vi "LIDAR V6 FPGA Main.vi"() -> ()   [LabVIEW 2013]
uses:
  Controls/FPGA Nain State.ctl
  Controls/Scan Format Typedaf.ctl
  <vilib>/Platform/TimedLoop/XDataNode/timing_clust.ctl
  <vilib>/Platform/TimedLoop/XDataNode/nitl_modes.ctl
  <vilib>/Platform/TimedLoop/XDataNode/wakeup.ctl
  Controls/Algorithm State.ctl
  <instrlib>/_niInstr/DSP/v1/Shared/Public/IQ Data.ctl
  <vilib>/rvi/Emulation/niFpgaSctlEmulationGetInTimedLoop.vi
  <vilib>/rvi/Emulation/niFpgaEmulationReportErrorSimple.vi
  <vilib>/rvi/Emulation/niFpgaGetClockAttributes.vi
  <vilib>/rvi/FIFO/Fifo_Resource/nirvififoEmulationReadFpgaImpl.vi
  <vilib>/rvi/DataTransferAndStorage/Container/Common/niFpgaContainerGetUniqueNameForEmu.vi
  <vilib>/rvi/eio/common/nirviEmuTemplateMethod_errors.vi
  <vilib>/rvi/Emulation/niFpgaCriticalErrorInLSC.vi
  <vilib>/rvi/Emulation/niFpgaProcessEmulError.vi
  LIDAR V2 Globals.vi
  <vilib>/rvi/FIFO/Fifo_Resource/nirvififoEmulationWriteFpgaImpl.vi
  <instrlib>/_niInstr/DSP/v1/FPGA/Private/Fractional Decimator/Fractional Decimator - 1 spc - 2x oc.vi
  <vilib>/rvi/interface/RandomDataEmulation/nirviRandomDataFPGAFIFO.vi
  <vilib>/rvi/interface/RandomDataEmulation/niFpgaRandomDataHandleErrors.vi
  <vilib>/Platform/TimedLoop/XDataNode/XDataNode.xnode
  <vilib>/rvi/DataTransferAndStorage/Container/XNode/niFpgaContainer.xnode
  <vilib>/rvi/FIFO/Fifo_Resource/nirvififoEmulationRead.vi
  <vilib>/eio/EIONode/EIONode.xnode
  <vilib>/rvi/FIFO/Fifo_Resource/nirvififoEmulationWrite.vi
  <vilib>/rvi/FXPMathLib/FxpInterpret/XNode/nifxpmath_Interpret.xnode
  <vilib>/rvi/interface/RandomDataEmulation/nirviRandomDataFpgaReadWriteTemplate.vi
  <vilib>/Platform/TimedLoop/XDataNode/XDNodeRunTimeDep.lvlib
  <instrlib>/_niInstr/DSP/v1/FPGA/niInstr DSP v1 FPGA.lvlib
  <instrlib>/_niInstr/DSP/v1/Shared/niInstr DSP v1 Shared.lvlib
panel:
  out "AI 0":i16
  in  "delay":fxp<+/-,16,0>
  in  "output sample rate":fxp<+,48,1>=0.799994660000003 format="%#.10g"
  in  "MaxStartSample":u8
  in  "LedScanDebEn":bool
  in  "ActiveLedIndexDeb":u16
  in  "10thIndexDeb":u8
  in  "PulseUpClck":u16=3
  in  "PulseWaitClck":u16=40
  in  "AO Trig":bool
  in  "Devider":u8=3
  in  "PFI3":bool
  in  "PFI2":bool
  in  "User Command Commit":bool
  in  "User Command":u8
  out "User Command Idle":bool
  out "User Command Status":u8
  in  "User Data 0":u8
  in  "User Data 1":u8
  out "User Error":bool
  out "Configured?":bool
  in  "MemDebStart":u32
  in  "MemDebEnd":u32
  in  "ReadMemSel":bool
  in  "ReadMem":bool
  in  "NextLedEn":bool
  out "SimCoarsMaxIndex":u16
  out "SimFineMaxIndex":u16
  out "SimOut":i16
  out "SPI Idle":bool
  out "PLL Locked":bool
  in  "Clock":u8=1
  out "PLL Counter":i32
  in  "IO Module\\Apply Settings":bool
  out "LedAddress":u16
  in  "SingleCycle":bool
  in  "PulsePerLed":i16=199
  in  "ScanFormat":T1=enum."FullScanPerLed"
  in  "SamplingEnable":bool
  out "MainState":T2
  out "10thIndex":u8
  out "PulseIndex":i16
  in  "MemSel":bool
  in  "ActiveLedIndex":u16
  out "InitMem":bool
  out "PulseEnd":bool
  in  "SampPerPulse":u16=99
  out "IterReset":u16 format="%.0b"
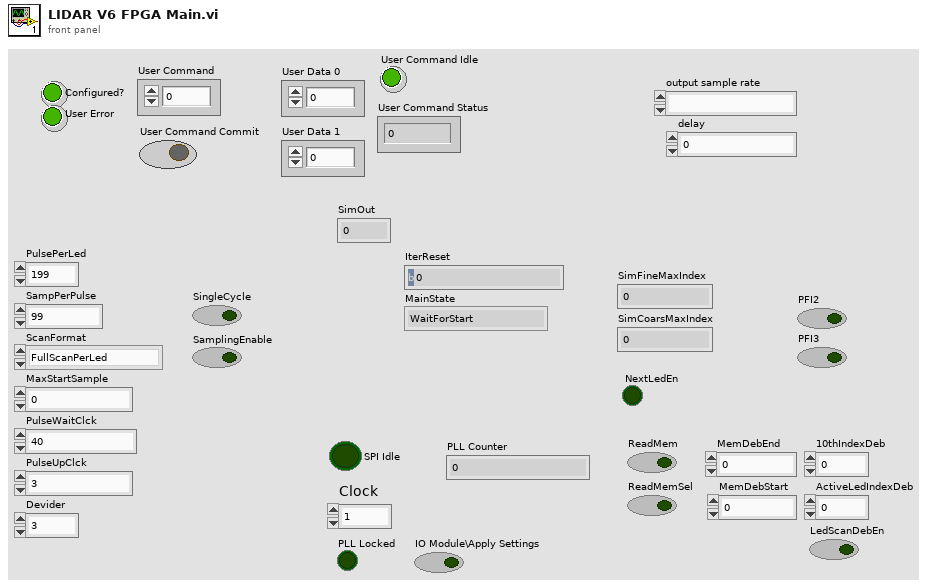
[diagram p1: front panel]
types:
  T1 = typedef "Scan Format Typedaf.ctl" = enum16{"1PulsePerLed", "FullScanPerLed"}
  T2 = typedef "FPGA Nain State.ctl" = enum16{"WaitForStart", "SetProcParams", "SelectActiveLed", "ActivatePulse", "WaitForPulseEnd", "WaitForAlgoStart", "SingleCycleEnd"}
  T3 = typedef "XDNodeRunTimeDep.lvlib/timing_clust.ctl" = cluster{"Expected End [f-1]":u64, "Actual End [f-1]":u64, "Finished Late? [f-1]":bool, "Expected End [i-1]":u64, "Actual End [i-1]":u64, "Finished Late? [i-1]":bool, "Expected Start [i]":u64, "Actual Start [i]":u64, "Expected Start [f]":u64, "Actual Start [f]":u64, "Source Name":string, "Structure Name":string, "Period":i64, "Deadline":i64, "Offset":i64, "Start":i64, "Priority":i32, "Timeout":i32, "Mode":T4, "Wakeup Reason":T5, "Error":errorcluster, "Source Type":string, "Secondary Source Type":string, "Global End Time":u64, "Global Start Time":u64, "Frame Duration":u64, "Iteration Duration":u64, "Assigned CPU":i32, "I/O Scan Engine Mode":u32}
  T4 = typedef "XDNodeRunTimeDep.lvlib/nitl_modes.ctl" = enum32{"No Change", "Process missed periods, maintain original phase", "Discard missed periods, maintain original phase", "Process missed periods, ignore original phase", "Discard missed periods, ignore original phase"}
  T5 = typedef "XDNodeRunTimeDep.lvlib/wakeup.ctl" = enum32{"Normal", "Aborted", "Asynchronous wakeup", "Timing source error", "Timed loop error", "Timeout"}
  T6 = typedef "niInstr DSP v1 Shared.lvlib/IQ Data.ctl" = cluster{"I":fxp<+/-,18,1>, "Q":fxp<+/-,18,1>, "overflow":bool}
  T7 = typedef "Algorithm State.ctl" = enum16{"WaitForStart", "GetNextSignalElement", "WaitForNextSignalElem", "MultWithSinc", "CalcMax"}
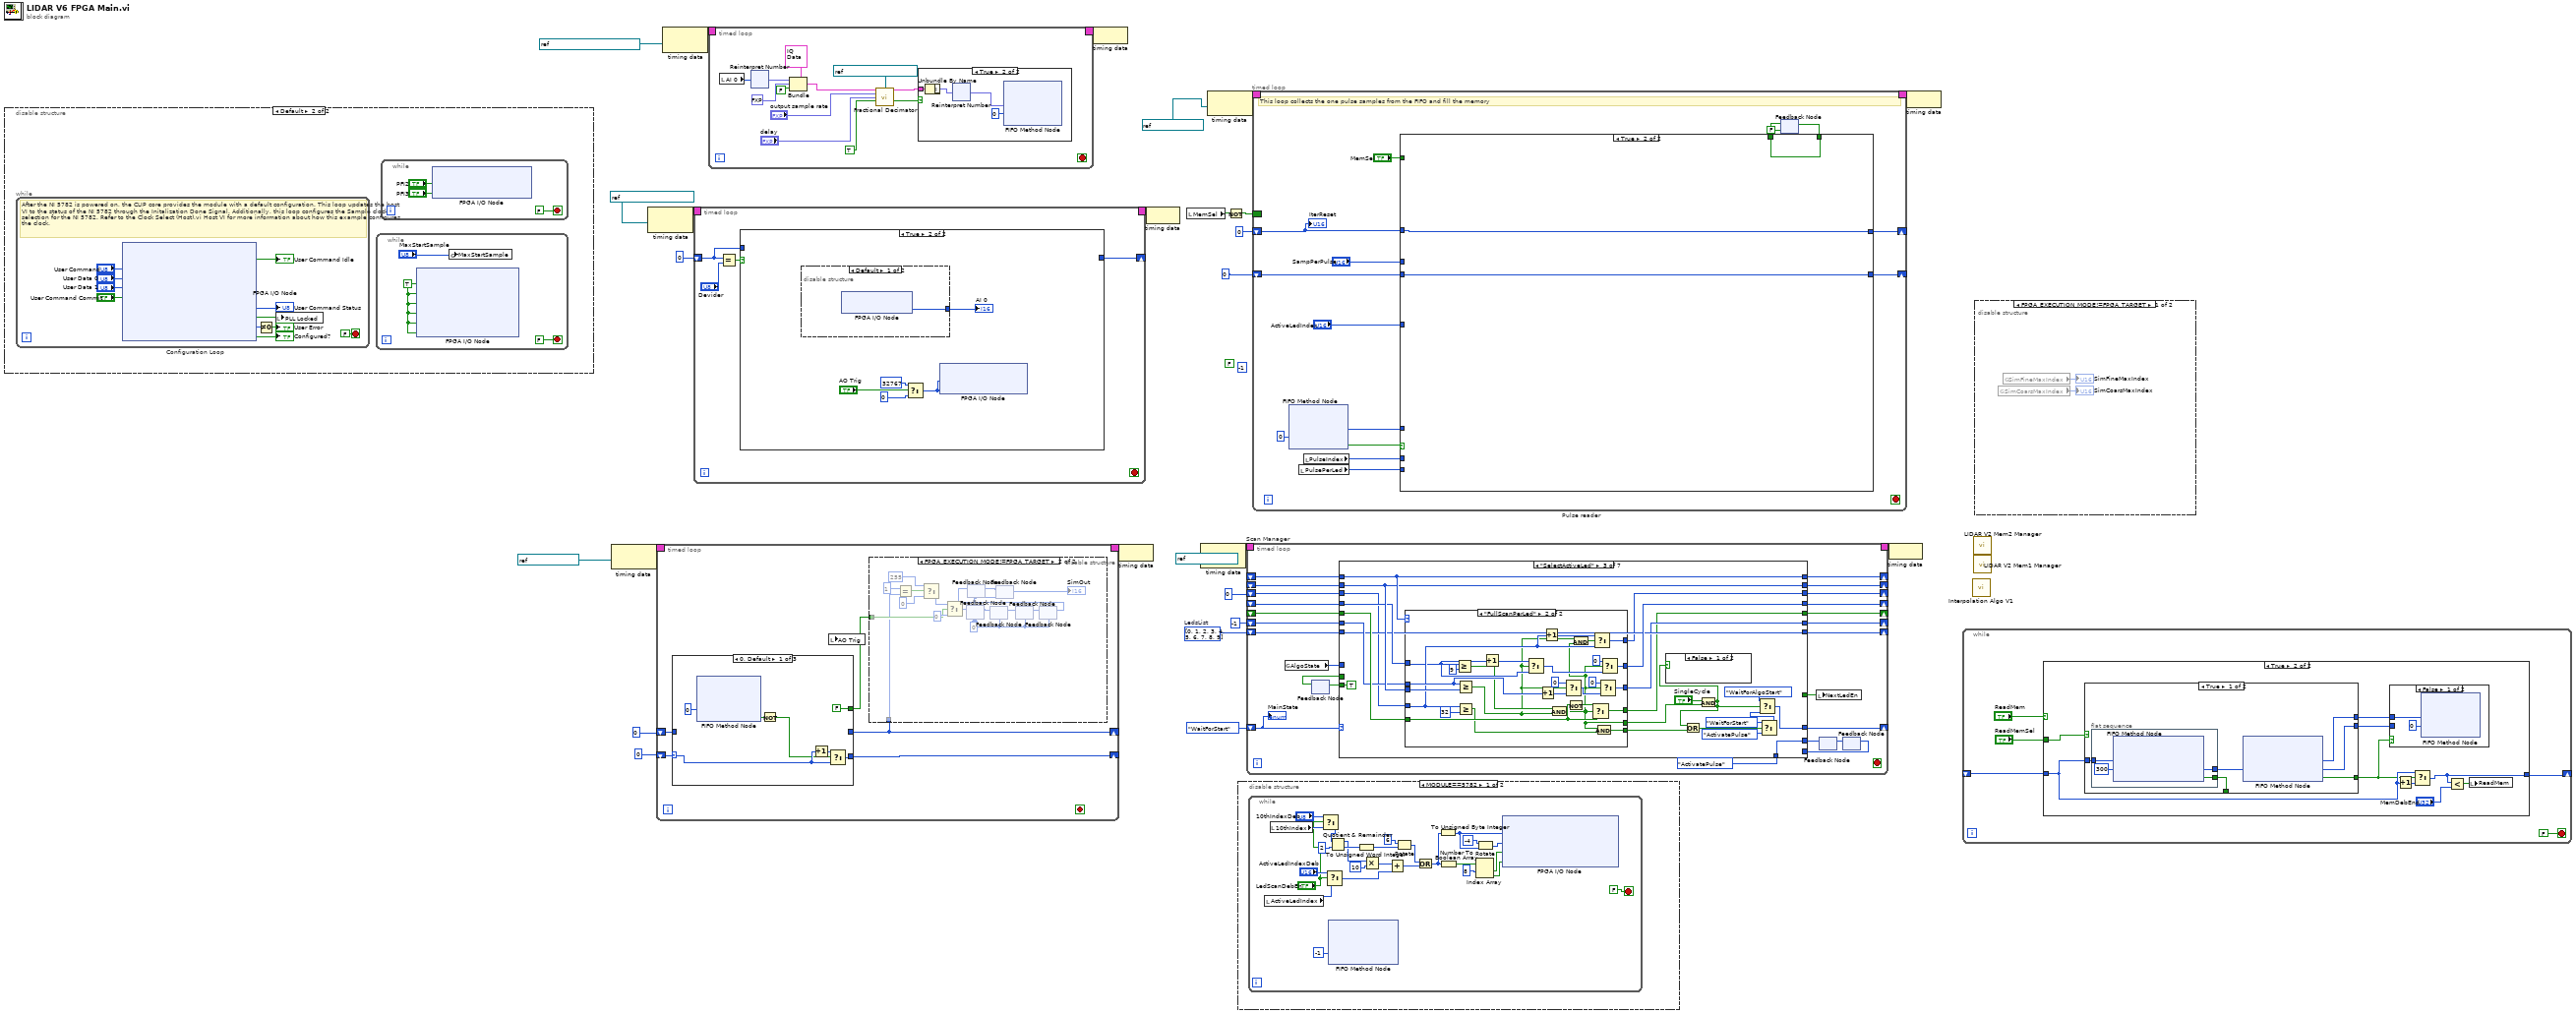
[diagram p0: block diagram]
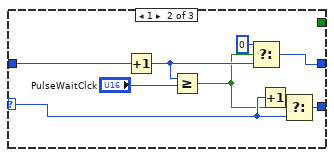
[diagram p4: hidden frame]
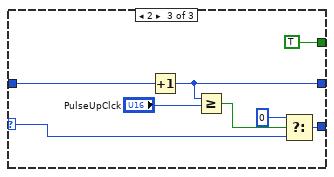
[diagram p5: hidden frame]
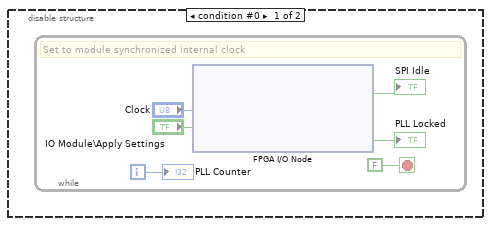
[diagram p7: hidden frame]
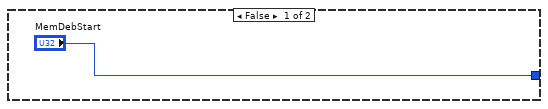
[diagram p8: hidden frame]
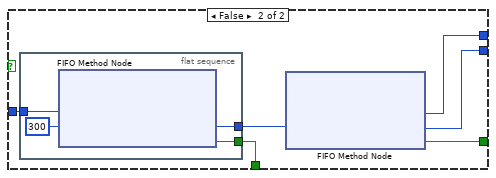
[diagram p10: hidden frame]
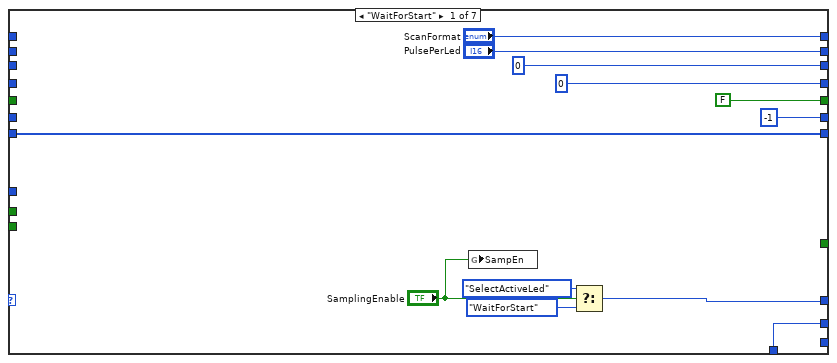
[diagram p12: hidden frame]
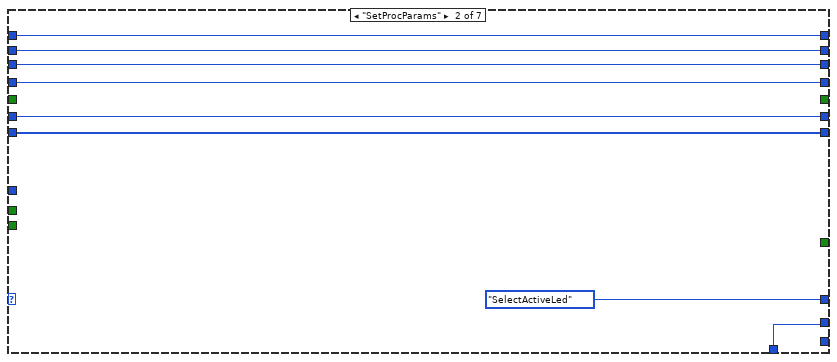
[diagram p13: hidden frame]
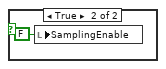
[diagram p14: hidden frame]
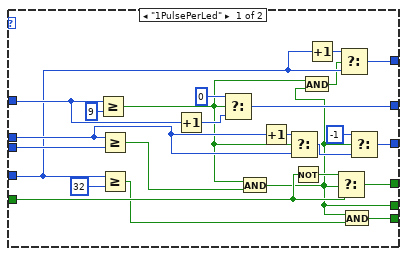
[diagram p15: hidden frame]
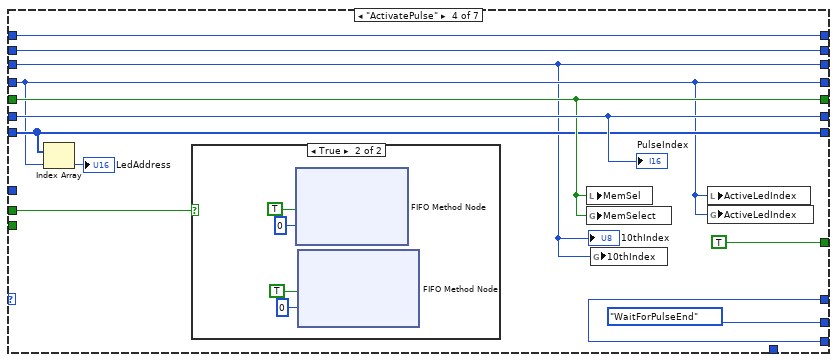
[diagram p16: hidden frame]
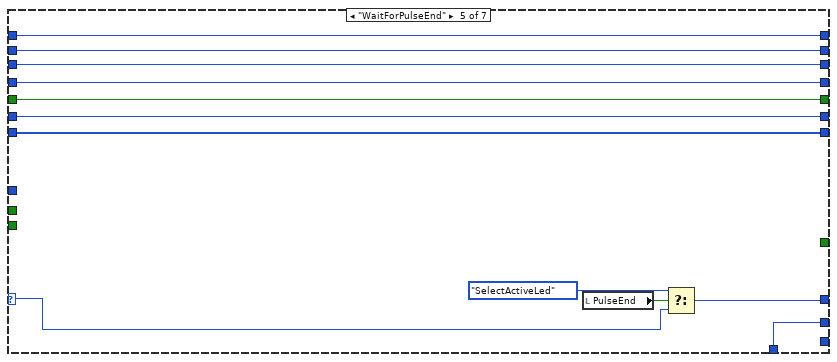
[diagram p18: hidden frame]
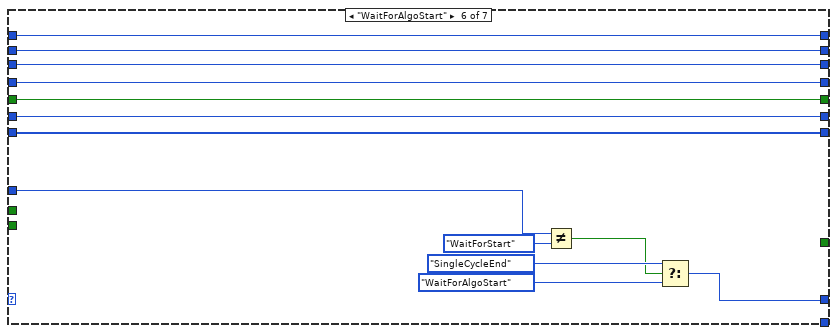
[diagram p19: hidden frame]
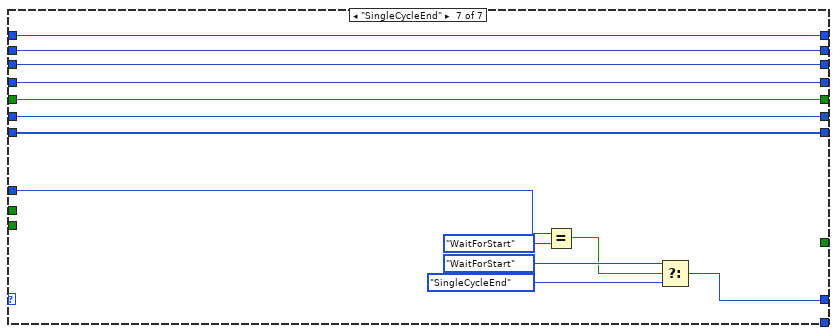
[diagram p20: hidden frame]
diagram:
  (unwired) FALSE
  w14 = u16[] [0, 1, 2, 3, 4, 5, 6, 7, 8, 9]  # LedsList
  (unwired) i16 -1 ("#Cycle")
  n1 = disable-structure shown="Default" {
    frame condition #0 {
      n2 = while {
        i -> [w29]
        stop <- FALSE stop-if-true
        # "Set to module synchronized internal clock"
        n3 = xnode "FPGA I/O Node"("IO Module\\Clock Select"="Clock", "IO Module\\Apply Settings"="IO Module\\Apply Settings") -> ("IO Module\\SPI Idle"=→"SPI Idle":bool, "IO Module\\PLL Locked"=→"PLL Locked":bool)  [unwired: 4 in, 4 out]
        "PLL Counter" <- w29
      }
    }
    frame condition #1 (active) {
      n4 = while "Configuration Loop" {
        stop <- FALSE stop-if-true
        # "After the NI 5782 is powered on, the CLIP core provides the module with a default configuration. This loop updates the host VI to the status of the NI 5782 through the Initalization Done Signal. Additionally, this loop configures the Sample clock selection for the NI 5782. Refer to the Clock Select (Host).vi Host VI for more information about how this example configures the clock."
        n5 = xnode "FPGA I/O Node"("IO Module\\User Command"="User Command", "IO Module\\User Data 0"="User Data 0", "IO Module\\User Data 1"="User Data 1", "IO Module\\User Command Commit"="User Command Commit") -> ("IO Module\\User Command Idle"=→"User Command Idle":bool, "IO Module\\User Command Status"=→"User Command Status":u8, "IO Module\\PLL Locked"=w36:bool, "IO Module\\User Error"=w40:u8, "IO Module\\Initialization Done"=→"Configured?":bool)  [unwired: 9 in, 9 out]
        n6 = Not Equal To 0?(x=w40) -> (x != 0?=→"User Error":bool)
        n7 = local write "PLL Locked"(w36) -> ()
      }
      n8 = while {
        stop <- FALSE stop-if-true
        w48 = TRUE ("IO Module\\DIO Port 0 WE")
        n9 = xnode "FPGA I/O Node"("IO Module\\DIO Port 0 WE"=w48, "IO Module\\DIO Port 1 WE"=w48, "IO Module\\PFI 0 WE"=w48, "IO Module\\PFI 1 WE"=w48, "IO Module\\PFI 2 WE"=w48, "IO Module\\PFI 3 WE"=w48) -> ()  [unwired: 6 in, 6 out]
        n10 = global write "LIDAR V2 Globals.vi" "MaxStartSample"("MaxStartSample") -> ()
      }
      n11 = while {
        stop <- FALSE stop-if-true
        n12 = xnode "FPGA I/O Node"("IO Module\\PFI 2 Wr Data"="PFI2", "IO Module\\PFI 3 Wr Data"="PFI3") -> ()  [unwired: 2 in, 2 out]
      }
    }
  }
  n13 = node-c288(refnum<k21> "100 MHz Clock" ("Source Name")) -> (w8:T3)
  n14 = node-c288(refnum<k21> "IO Module\\Data Clock" ("Source Name")) -> (w26:T3)
  n15 = timed-loop {
    timing: w8 -> [_]
    timing-out: [_] -> w7
    shift-right: [w53] -> _
    shift-left: i16 0 -> [w54]
    shift-right: [w51] -> _
    shift-left: u16 0 -> [w52]
    stop <- _ stop-if-true
    n16 = case shown="0, Default" w54 {
      selector: w54 -> [w76 w83 w89]
      tunnel: [w77 w84 w90] -> w53
      tunnel: w52 -> [_ w86 w94]
      tunnel: [_ w80 w93] -> w51
      tunnel: [FALSE _ TRUE] -> w50
      frame 0, Default {
        n17 = xnode ("FIFO Method Node")("Timeout"=0) -> ("Timed Out?"=w73:bool)  [unwired: 1 in, 2 out]
        n18 = Not(x=w73) -> (.not. x?=w71:bool)
        n19 = Increment(x=w76) -> (x+1=w75:i16)
        n20 = Select(t=w75, s=w71, f=w76) -> (s? t:f=w77:i16)
      }
      frame 1 {
        n21 = Increment(x=w86) -> (x+1=w81:u16)
        n22 = Greater Or Equal?(x=w81, y="PulseWaitClck") -> (x >= y?=w78:bool)
        n23 = Select(t=u16 0, s=w78, f=w81) -> (s? t:f=w80:u16)
        n24 = Increment(x=w83) -> (x+1=w82:i16)
        n25 = Select(t=w82, s=w78, f=w83) -> (s? t:f=w84:i16)
      }
      frame 2 {
        n26 = Increment(x=w94) -> (x+1=w93:u16)
        n27 = Greater Or Equal?(x=w93, y="PulseUpClck") -> (x >= y?=w91:bool)
        n28 = Select(t=i16 0, s=w91, f=w89) -> (s? t:f=w90:i16)
      }
    }
    n29 = local write "AO Trig"(w50) -> ()
    n30 = disable-structure shown="FPGA_EXECUTION_MODE!=FPGA_TARGET" {
      disable-tunnel: w50 -> [_ w62]
      disable-tunnel: w51 -> [_ w61]
      frame condition #0 (active) {
      }
      frame condition #1 {
        w65 = i16 0 ("IO Module\\AO 0")
        n31 = Equal?(x=u16 1, y=w61) -> (x = y?=w59:bool)
        n32 = Select(t=i16 255 ("IO Module\\AO 0"), s=w59, f=i16 0) -> (s? t:f=w60:i16)
        n33 = Select(t=w60, s=w62, f=i16 0 ("IO Module\\AO 0")) -> (s? t:f=w63:i16)
        n34 = feedback-in #1(w63) -> ()
        n35 = feedback #1(w65) -> (w70:i16)
        n36 = feedback #2(w65) -> (w66:i16)
        n37 = feedback #3(w65) -> (w69:i16)
        n38 = feedback-in #3(w70) -> ()
        n39 = feedback #4(w65) -> (→"SimOut":i16)
        n40 = feedback-in #4(w66) -> ()
        n41 = feedback #5(w65) -> (w68:i16)
        n42 = feedback-in #5(w69) -> ()
        n43 = feedback #6(w65) -> (w67:i16)
        n44 = feedback-in #2(w67) -> ()
        n45 = feedback-in #6(w68) -> ()
      }
    }
  }
  n46 = node-c288(refnum<k21> "IO Module\\Data Clock Div 2" ("Source Name")) -> (w3:T3)
  n47 = timed-loop {
    timing: w26 -> [_]
    timing-out: [_] -> w25
    shift-right: [w97] -> _
    shift-left: u8 0 -> [w98]
    stop <- _ stop-if-true
    n48 = Equal?(x=w98, y="Devider") -> (x = y?=w99:bool)
    n49 = case shown="True" w99 {
      tunnel: w98 -> [w102 _]
      tunnel: [w101 _] -> w97
      frame False {
        n50 = Increment(x=w102) -> (x+1=w101:u8)
      }
      frame True {
        n51 = disable-structure shown="Default" {
          disable-tunnel: [w108 w109] -> w107
          frame condition #0 (active) {
            n52 = xnode "FPGA I/O Node"() -> ("IO Module\\AI 0"=w108:i16)  [unwired: 1 in, 1 out]
          }
          frame condition #1 {
            n53 = local read "SimOut"() -> (w109:i16)
          }
        }
        "AI 0" <- w107
        n54 = Select(t=i16 32767 ("IO Module\\AO 0"), s="AO Trig", f=i16 0 ("IO Module\\AO 0")) -> (s? t:f=w106:i16)
        n55 = xnode "FPGA I/O Node"("IO Module\\AO 0 N-1"=w106, "IO Module\\AO 0 N"=w106) -> ()  [unwired: 2 in, 2 out]
      }
    }
  }
  n56 = timed-loop {
    timing: w3 -> [_]
    timing-out: [_] -> w2
    stop <- _ stop-if-true
    n57 = local read "AI 0"() -> (w115:i16)
    n58 = xnode "Reinterpret Number"("x"=w115) -> ("y"=w121:fxp<+/-,16,1>)
    n59 = Bundle(cluster=T6 {"I"=0.0, "Q"=0.0, "overflow"=FALSE} ("data in"), "I"=w121, "Q"=fxp<+/-,18,1> 0.0, "overflow"=FALSE) -> (w116:T6)
    n60 = call-poly <instrlib>:"Fractional Decimator.vi"("data in"=w116, "clock x 2"=refnum<k21> "IO Module\\Data Clock", "output sample rate"="output sample rate", "delay"="delay", "input valid"=TRUE) -> ("data out"=w114:T6, "output valid"=w113:bool)  [unwired: 8 in, 1 out]
    n61 = case shown="True" w113 {
      tunnel: w114 -> [_ w125]
      frame False {
      }
      frame True {
        n62 = Unbundle By Name(w125) -> ("I"=w126:fxp<+/-,18,1>)
        n63 = xnode "Reinterpret Number"("x"=w126) -> ("y"=w124:fxp<+/-,18,16>)
        n64 = xnode ("FIFO Method Node")("Element"=w124, "Timeout"=0) -> ()  [unwired: 1 in, 2 out]
      }
    }
  }
  n65 = node-c288(w2) -> ()
  n66 = node-c288(w7) -> ()
  n67 = node-c288(w25) -> ()
  n68 = local read "MemSel"() -> (w19:bool)
  n69 = node-c288(refnum<k21> "100 MHz Clock" ("Source Name")) -> (w22:T3)
  n70 = node-c288(refnum<k21> "100 MHz Clock" ("Source Name")) -> (w24:T3)
  n71 = Not(x=w19) -> (.not. x?=w18:bool)
  n72 = disable-structure shown="MODULE==5782" {
    frame condition #0 (active) {
      n73 = while {
        stop <- FALSE stop-if-true
        n74 = local read "ActiveLedIndex"() -> (w134:u16)
        n75 = local read "10thIndex"() -> (w136:u8)
        n76 = Select(t="10thIndexDeb", s="LedScanDebEn", f=w136) -> (s? t:f=w135:u8)
        n77 = Select(t="ActiveLedIndexDeb", s="LedScanDebEn", f=w134) -> (s? t:f=w133:u16)
        n78 = xnode ("FIFO Method Node")("Timeout"=-1) -> ()  [unwired: 1 in, 3 out]
        n79 = Quotient & Remainder(x=w135, y=u8 2) -> (x-y*floor(x/y)=w140:u8, floor(x/y)=w141:u8)
        n80 = To Unsigned Word Integer(number=w141) -> (unsigned 16bit integer=w148:u16)
        n81 = Multiply(x=w140, y=u8 10) -> (x*y=w139:u8)
        n82 = Add(x=w139, y=w133) -> (x+y=w154:u16)
        n83 = Rotate(1:w148, 2:u16 6 ("x")) -> (0:w155:u16)
        n84 = Or(x=w155, y=w154) -> (x .or. y?=w153:u16)
        n85 = To Unsigned Byte Integer(number=w153) -> (unsigned 8bit integer=w145:u8)
        n86 = Number To Boolean Array(number=w153) -> (Boolean array=w152:bool[])
        n87 = Index Array(array=w152, index #1=8 ("index")) -> (element #1=w150:bool, element #2=w149:bool)  [unwired: 1 in]
        n88 = Rotate(1:w145, 2:i16 -4 ("y")) -> (0:w143:u8)
        n89 = xnode "FPGA I/O Node"("IO Module\\DIO Port 0 Wr Data"=w145, "IO Module\\DIO Port 1 Wr Data"=w143, "IO Module\\PFI 0 Wr Data"=w150, "IO Module\\PFI 1 Wr Data"=w149) -> ()  [unwired: 4 in, 4 out]
      }
    }
    frame condition #1 {
    }
  }
  n90 = timed-loop "Scan Manager" {
    timing: w22 -> [_]
    timing-out: [_] -> w21
    shift-right: [w178] -> _
    shift-left: FPGA_Nain_State."WaitForStart" ("MainState") -> [w179]
    shift-right: [w177] -> _
    shift-left: _ -> [w175]
    shift-right: [w176] -> _
    shift-left: _ -> [w174]
    shift-right: [w167] -> _
    shift-left: u8 0 ("10thIndex") -> [w173]
    shift-right: [w157] -> _
    shift-left: _ -> [w172]
    shift-right: [w161] -> _
    shift-left: _ -> [w171]
    shift-right: [w170] -> _
    shift-left: i16 -1 -> [w160]
    shift-right: [w168] -> _
    shift-left: w14 -> [w169]
    stop <- _ stop-if-true
    n91 = global read "LIDAR V2 Globals.vi" "AlgoState"() -> (w156:T7)
    n92 = feedback #7() -> (w158:bool)  [unwired: 1 in]
    n93 = feedback #8() -> (w164:T2)  [unwired: 1 in]
    n94 = feedback #9() -> (w163:T2)  [unwired: 1 in]
    n95 = case shown="\"SelectActiveLed\"" w179 {
      selector: w179 -> [_ _ _ _ w295 _ _]
      tunnel: [w189 FPGA_Nain_State."SelectActiveLed" ("MainState") w203 w281 w294 w305 w318] -> w178
      tunnel: ["ScanFormat" w195 w222 w285 w301 w314 w327] -> w177
      tunnel: ["PulsePerLed" w194 w220 w284 w300 w313 w326] -> w176
      tunnel: w175 -> [_ w195 w222 w285 w301 w314 w327]
      tunnel: w174 -> [_ w194 w220 w284 w300 w313 w326]
      tunnel: [u8 0 ("10thIndex") w193 w211 w274 w299 w312 w325] -> w167
      tunnel: w173 -> [_ w193 w212 w274 w299 w312 w325]
      tunnel: [u16 0 ("ActiveLedIndex") w192 w217 w275 w298 w311 w324] -> w157
      tunnel: w172 -> [_ w192 w218 w275 w298 w311 w324]
      tunnel: [FALSE _ w214 w278 w297 w310 w323] -> w161
      tunnel: w171 -> [_ _ w221 w278 w297 w310 w323]
      tunnel: [i16 -1 ("t") w198 w215 w279 w292 w309 w322] -> w170
      tunnel: w160 -> [_ w198 w219 w279 w292 w309 w322]
      tunnel: w169 -> [w187 w197 w216 w276 w291 w308 w321]
      tunnel: [w187 w197 w216 w276 w291 w308 w321] -> w168
      tunnel: [_ _ _ TRUE ("SampEnable") _ _ _] -> w166
      tunnel: [w186 w196 w210 FPGA_Nain_State."WaitForPulseEnd" ("MainState") w290 _ _] -> w165
      tunnel: w163 -> [_ _ _ w281 _ _ _]
      tunnel: FPGA_Nain_State."ActivatePulse" ("MainState") -> [w186 w196 w210 _ w290 _ _]
      tunnel: [_ _ TRUE _ _ _ _] -> w159
      tunnel: w158 -> [_ _ _ w280 _ _ _]
      tunnel: w156 -> [_ _ _ _ _ w302 w316]
      frame "WaitForStart" {
        n96 = global write "LIDAR V2 Globals.vi" "SampEn"("SamplingEnable") -> ()
        n97 = Select(t=FPGA_Nain_State."SelectActiveLed" ("MainState"), s="SamplingEnable", f=FPGA_Nain_State."WaitForStart" ("MainState")) -> (s? t:f=w189:T2)
      }
      frame "SetProcParams" {
      }
      frame "SelectActiveLed" {
        n98 = case shown="\"FullScanPerLed\"" w222 {
          tunnel: w221 -> [w239 w269]
          tunnel: w212 -> [w232 w264]
          tunnel: w220 -> [w242 w271]
          tunnel: w218 -> [w245 w255]
          tunnel: w219 -> [w241 w270]
          tunnel: [w233 w251] -> w217
          tunnel: [w228 w253] -> w215
          tunnel: [w236 w267] -> w214
          tunnel: [w234 w265] -> w208
          tunnel: [w230 w262] -> w211
          tunnel: [w224 w248] -> w209
          frame "1PulsePerLed" {
            n99 = Greater Or Equal?(x=w245, y=u16 9) -> (x >= y?=w226:bool)
            n100 = Greater Or Equal?(x=w241, y=w242) -> (x >= y?=w237:bool)
            n101 = Greater Or Equal?(x=w232, y=u8 32) -> (x >= y?=w235:bool)
            n102 = Increment(x=w245) -> (x+1=w244:u16)
            n103 = Select(t=u16 0, s=w226, f=w244) -> (s? t:f=w233:u16)
            n104 = And(x=w226, y=w237) -> (x .and. y?=w224:bool)
            n105 = Increment(x=w241) -> (x+1=w240:i16)
            n106 = Select(t=w240, s=w226, f=w241) -> (s? t:f=w229:i16)
            n107 = Not(x=w239) -> (.not. x?=w238:bool)
            n108 = And(x=w226, y=w224) -> (x .and. y?=w225:bool)
            n109 = Increment(x=w232) -> (x+1=w231:u8)
            n110 = Select(t=w238, s=w224, f=w239) -> (s? t:f=w236:bool)
            n111 = Select(t=w231, s=w225, f=w232) -> (s? t:f=w230:u8)
            n112 = And(x=w224, y=w235) -> (x .and. y?=w234:bool)
            n113 = Select(t=i16 -1, s=w224, f=w229) -> (s? t:f=w228:i16)
          }
          frame "FullScanPerLed" {
            n114 = Greater Or Equal?(x=w255, y=u16 9) -> (x >= y?=w254:bool)
            n115 = Greater Or Equal?(x=w270, y=w271) -> (x >= y?=w249:bool)
            n116 = Greater Or Equal?(x=w264, y=u8 32) -> (x >= y?=w266:bool)
            n117 = Increment(x=w255) -> (x+1=w256:u16)
            n118 = Select(t=w256, s=w249, f=w255) -> (s? t:f=w252:u16)
            n119 = Increment(x=w270) -> (x+1=w258:i16)
            n120 = Increment(x=w264) -> (x+1=w263:u8)
            n121 = And(x=w254, y=w249) -> (x .and. y?=w248:bool)
            n122 = Select(t=i16 0, s=w249, f=w258) -> (s? t:f=w261:i16)
            n123 = Not(x=w269) -> (.not. x?=w268:bool)
            n124 = And(x=w249, y=w248) -> (x .and. y?=w259:bool)
            n125 = Select(t=w268, s=w248, f=w269) -> (s? t:f=w267:bool)
            n126 = Select(t=w263, s=w259, f=w264) -> (s? t:f=w262:u8)
            n127 = And(x=w248, y=w266) -> (x .and. y?=w265:bool)
            n128 = Select(t=i16 0, s=w248, f=w261) -> (s? t:f=w253:i16)
            n129 = Select(t=u16 0, s=w248, f=w252) -> (s? t:f=w251:u16)
          }
        }
        n130 = And(x="SingleCycle", y=w209) -> (x .and. y?=w200:bool)
        n131 = case shown="False" w200 {
          frame False {
          }
          frame True {
            n132 = local write "SamplingEnable"(FALSE ("SamplingEnable")) -> ()
          }
        }
        n133 = Or(x=w200, y=w208) -> (x .or. y?=w207:bool)
        n134 = Select(t=FPGA_Nain_State."WaitForStart" ("MainState"), s=w207, f=FPGA_Nain_State."ActivatePulse" ("MainState")) -> (s? t:f=w204:T2)
        n135 = Select(t=FPGA_Nain_State."WaitForAlgoStart" ("MainState"), s=w200, f=w204) -> (s? t:f=w203:T2)
      }
      frame "ActivatePulse" {
        n136 = Index Array(array=w276, index=w275) -> (element=→"LedAddress":u16)
        n137 = case shown="True" w280 {
          frame False {
          }
          frame True {
            n138 = xnode ("FIFO Method Node")("Element"=TRUE ("GenPulse"), "Timeout"=0) -> ()  [unwired: 1 in, 2 out]
            n139 = xnode ("FIFO Method Node")("Element"=TRUE ("GenPulse"), "Timeout"=0) -> ()  [unwired: 1 in, 2 out]
          }
        }
        n140 = local write "MemSel"(w278) -> ()
        n141 = global write "LIDAR V2 Globals.vi" "MemSelect"(w278) -> ()
        n142 = global write "LIDAR V2 Globals.vi" "10thIndex"(w274) -> ()
        n143 = local write "ActiveLedIndex"(w275) -> ()
        n144 = global write "LIDAR V2 Globals.vi" "ActiveLedIndex"(w275) -> ()
        "PulseIndex" <- w279
        "10thIndex" <- w274
      }
      frame "WaitForPulseEnd" {
        n145 = local read "PulseEnd"() -> (w296:bool)
        n146 = Select(t=FPGA_Nain_State."SelectActiveLed", s=w296, f=w295) -> (s? t:f=w294:T2)
      }
      frame "WaitForAlgoStart" {
        n147 = Not Equal?(x=w302, y=Algorithm_State."WaitForStart") -> (x != y?=w303:bool)
        n148 = Select(t=FPGA_Nain_State."SingleCycleEnd", s=w303, f=FPGA_Nain_State."WaitForAlgoStart" ("MainState")) -> (s? t:f=w305:T2)
      }
      frame "SingleCycleEnd" {
        n149 = Equal?(x=w316, y=Algorithm_State."WaitForStart") -> (x = y?=w315:bool)
        n150 = Select(t=FPGA_Nain_State."WaitForStart", s=w315, f=FPGA_Nain_State."SingleCycleEnd" ("MainState")) -> (s? t:f=w318:T2)
      }
    }
    n151 = feedback-in #7(w159) -> ()
    n152 = local write "NextLedEn"(w166) -> ()
    n153 = feedback-in #8(w165) -> ()
    n154 = feedback-in #9(w164) -> ()
    "MainState" <- w179
  }
  n155 = timed-loop "Pulse reader" {
    timing: w24 -> [_]
    timing-out: [_] -> w23
    shift-right: [w341] -> _
    shift-left: u16 0 -> [w339]
    border: w18 -> [_]
    shift-right: [w331] -> _
    shift-left: u16 0 -> [w330]
    stop <- _ stop-if-true
    # "This loop collects the one pulse samples from the FIFO and fill the memory"
    n156 = xnode ("FIFO Method Node")("Timeout"=0) -> ("Element"=w343:i16, "Timed Out?"=w342:bool)  [unwired: 1 in, 1 out]
    n157 = local read "PulsePerLed"() -> (w332:i16)
    n158 = local read "PulseIndex"() -> (w333:i16)
    n159 = feedback #10(FALSE) -> (w337:bool)
    n160 = case shown="True" w342 {
      tunnel: w343 -> [w395 _]
      tunnel: "ActiveLedIndex" -> [w348 _]
      tunnel: "SampPerPulse" -> [w394 _]
      tunnel: [w374 w406] -> w341
      tunnel: w339 -> [w396 w406]
      tunnel: [w353 w405] -> w338
      tunnel: w337 -> [w352 w405]
      tunnel: "MemSel" -> [w366 _]
      tunnel: w333 -> [w392 _]
      tunnel: w332 -> [w391 _]
      tunnel: [w346 w404] -> w331
      tunnel: w330 -> [w345 w404]
      frame False {
        w384 = u16 16384  # LastIterration
        w350 = u16 32768  # FirstIterration
        n161 = feedback #11() -> (w398:bool)
        n162 = feedback-in #11(w366) -> ()
        n163 = Greater Or Equal?(x=w345, y=w394) -> (x >= y?=w355:bool)
        "PulseEnd" <- w355
        n164 = Equal?(x=w392, y=w391) -> (x = y?=w393:bool)
        n165 = Not Equal?(x=w366, y=w398) -> (x != y?=w399:bool)
        n166 = Select(t=u16 0, s=w399, f=w396) -> (s? t:f=w351:u16)
        n167 = Multiply(x=w348, y=u16 100) -> (x*y=w389:u16)
        n168 = And(x=w348, y=u16 15) -> (x .and. y?=w380:u16)
        n169 = Add(x=w389, y=w345) -> (x+y=w388:u16)
        n170 = To Word Integer(number=w348) -> (16bit integer=w360:i16)
        n171 = Select(t=u16 0 ("x"), s=w352, f=w350) -> (s? t:f=w387:u16)
        n172 = Select(t=w384, s=w393, f=u16 0 ("x")) -> (s? t:f=w383:u16)
        n173 = Negate(x=w360) -> (-x=w356:i16)
        n174 = Or(x=w387, y=w388) -> (x .or. y?=w382:u16)
        n175 = Or(x=w382, y=w383) -> (x .or. y?=w377:u16)
        n176 = Rotate(1:w380, 2:i16 10 ("y")) -> (0:w378:u16)
        n177 = Or(x=w377, y=w378) -> (x .or. y?=w376:u16)
        n178 = Select(t=i16 2, s=w366, f=i16 0) -> (s? t:f=w362:i16)
        n179 = Select(t=i16 0, s=w355, f=i16 1) -> (s? t:f=w361:i16)
        n180 = Rotate(1:w351, 2:w356) -> (0:w357:u16)
        n181 = Logical Shift(y=w348, x=u16 1) -> (x << y=w371:u16)
        n182 = Join Numbers(hi=w395, lo=w376) -> ((hi.lo)=w386:u32)
        n183 = And(x=u16 1, y=w357) -> (x .and. y?=w359:u16)
        n184 = Or(x=w361, y=w362) -> (x .or. y?=w363:i16)
        n185 = Greater Than 0?(x=w359) -> (x > 0?=w354:bool)
        n186 = Or(x=w351, y=w371) -> (x .or. y?=w369:u16)
        n187 = case shown="1" w363 {
          tunnel: w386 -> [w400 w402 _]
          frame 1 {
            n188 = xnode ("FIFO Method Node")("Element"=w400, "Timeout"=0) -> ()  [unwired: 1 in, 2 out]
          }
          frame 3 {
            n189 = xnode ("FIFO Method Node")("Element"=w402, "Timeout"=0) -> ()  [unwired: 1 in, 2 out]
          }
          frame Default {
          }
        }
        n190 = Increment(x=w345) -> (x+1=w375:u16)
        n191 = Select(t=w345, s=w355, f=w375) -> (s? t:f=w347:u16)
        n192 = Select(t=w369, s=w355, f=w351) -> (s? t:f=w374:u16)
        n193 = Select(t=w354, s=w355, f=w352) -> (s? t:f=w353:bool)
        "InitMem" <- w353
        n194 = Select(t=u16 0, s="NextLedEn", f=w347) -> (s? t:f=w346:u16)
      }
      frame True {
      }
    }
    n195 = feedback-in #10(w338) -> ()
    "IterReset" <- w339
  }
  n196 = node-c288(w21) -> ()
  n197 = node-c288(w23) -> ()
  n198 = while {
    shift-right: [w411] -> _
    shift-left: _ -> [w410]
    stop <- FALSE stop-if-true
    n199 = case shown="True" "ReadMem" {
      tunnel: "ReadMemSel" -> [_ w418]
      tunnel: ["MemDebStart" w421] -> w411
      tunnel: w410 -> [_ w423]
      frame False {
      }
      frame True {
        n200 = case shown="True" w418 {
          tunnel: w423 -> [w430 w438]
          tunnel: [w429 w437] -> w415
          tunnel: [w428 w436] -> w417
          tunnel: [w427 w435] -> w416
          tunnel: [w426 w434] -> _
          frame True {
            n201 = flat-sequence {
              tunnel: w430 -> [w433]
              tunnel: [w432] -> w427
              tunnel: [w431] -> w426
              frame #0 {
                w432 = 300 ("Timeout")
                n202 = xnode ("FIFO Method Node")("Element"=w433, "Timeout"=w432) -> ("Timed Out?"=w431:bool)  [unwired: 1 in, 1 out]
              }
            }
            n203 = xnode ("FIFO Method Node")("Timeout"=w427) -> ("Element"=w428:u64, "Timed Out?"=w429:bool)  [unwired: 1 in, 1 out]
          }
          frame False {
            n204 = flat-sequence {
              tunnel: w438 -> [w441]
              tunnel: [w440] -> w435
              tunnel: [w439] -> w434
              frame #0 {
                w440 = 300 ("Timeout")
                n205 = xnode ("FIFO Method Node")("Element"=w441, "Timeout"=w440) -> ("Timed Out?"=w439:bool)  [unwired: 1 in, 1 out]
              }
            }
            n206 = xnode ("FIFO Method Node")("Timeout"=w435) -> ("Element"=w436:u64, "Timed Out?"=w437:bool)  [unwired: 1 in, 1 out]
          }
        }
        n207 = case shown="False" w415 {
          tunnel: w417 -> [w425 _]
          tunnel: w416 -> [_ _]
          frame False {
            n208 = xnode ("FIFO Method Node")("Element"=w425, "Timeout"=0) -> ()  [unwired: 1 in, 2 out]
          }
          frame True {
          }
        }
        n209 = Increment(x=w423) -> (x+1=w422:u32)
        n210 = Select(t=w423, s=w415, f=w422) -> (s? t:f=w421:u32)
        n211 = Less?(x=w421, y="MemDebEnd") -> (x < y?=w419:bool)
        n212 = local write "ReadMem"(w419) -> ()
      }
    }
  }
  n213 = call "Interpolation Algo V1.vi"() -> ()  [unwired: 10 in, 2 out]
  n214 = call "LIDAR V2 Mem2 Manager.vi"() -> ()  [unwired: 12 in]
  n215 = call "LIDAR V2 Mem1 Manager.vi"() -> ()  [unwired: 12 in]
  n216 = disable-structure shown="FPGA_EXECUTION_MODE!=FPGA_TARGET" {
    frame condition #0 {
      n217 = global read "LIDAR V2 Globals.vi" "SimCoarsMaxIndex"() -> (→"SimCoarsMaxIndex":u16)
      n218 = global read "LIDAR V2 Globals.vi" "SimFineMaxIndex"() -> (→"SimFineMaxIndex":u16)
    }
    frame condition #1 (active) {
    }
  }
